vi "PowU64.vi"(4 "y":u64, 5 "x":u64) -> (1 "x^y":u64, 2 "Overflow?":bool)   [LabVIEW 2017, in "GPOverflow.lvlib"]
doc: "Computes <B>x</B> to the <B>y</B>'th power keeping track of numeric overflow.\n\n<B>Overflow?</B> will be True if positive or negative overflow occurred. The output will saturate in case of overflow.\n\nThis VI is inlined.\n\nSteen Schmidt\nGPower\n8/8 2013"
uses:
  GPOverflow.lvlib
  Mult/MultU64.vi
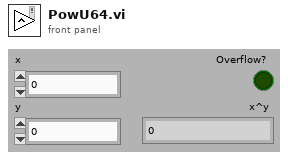
[diagram p1: front panel]
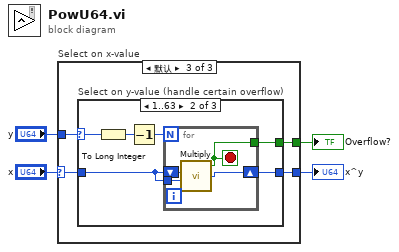
[diagram p0: block diagram]
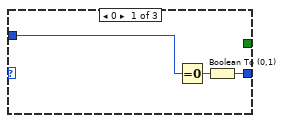
[diagram p2: hidden frame]
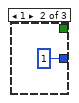
[diagram p3: hidden frame]
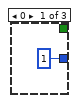
[diagram p4: hidden frame]
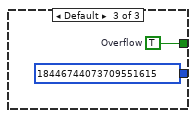
[diagram p5: hidden frame]
diagram:
  n1 = case "Select on x-value" shown="默认" "x" {
    selector: "x" -> [_ _ w10]
    tunnel: [_ _ w12] -> w4
    tunnel: [w5 u64 1 ("x") w11] -> w3
    tunnel: "y" -> [w7 _ w9]
    frame 0 {
      n2 = Equal To 0?(x=w7) -> (x = 0?=w6:bool)
      n3 = Boolean To (0,1)(Boolean=w6) -> (0, 1=w5:i16)
    }
    frame 1 {
    }
    frame Default {
      n4 = case "Select on y-value (handle certain overflow)" shown="1..63" w9 {
        selector: w9 -> [_ w14 _]
        tunnel: [_ w17 w25] -> w12
        tunnel: [u64 1 ("x") w16 u64 18446744073709551615 ("x")] -> w11
        tunnel: w10 -> [_ w15 _]
        frame 0 {
        }
        frame 1..63 {
          n5 = To Long Integer(number=w14) -> (32bit integer=w19:i32)
          n6 = Decrement(x=w19) -> (x-1=w18:i32)
          n7 = for {
            N: w18 -> [_]
            shift-right: [w21] -> w16
            shift-left: w15 -> [w23]
            tunnel: w15 -> [w22]
            tunnel: [w20] -> w17
            stop <- w20 stop-if-true
            n8 = call-poly "Multiply.vi"("y"=w22, "x"=w23) -> ("x*y"=w21:u64, "Overflow?"=w20:bool)  [unwired: 3 in]
          }
        }
        frame Default {
          w25 = TRUE  # Overflow
        }
      }
    }
  }
  "x^y" <- w3
  "Overflow?" <- w4
